vi "给选中行上色.vi"(4 "列数":i32, 6 "颜色":cluster{"未选中颜色盒":u32, "选中颜色盒":u32}={"未选中颜色盒"=16763272, "选中颜色盒"=12439011}, 8 "错误输入（无错误）":errorcluster, 9 "本次坐标":T1={"Row"=20, "Column"=20}, 10 "上次坐标":T1={"Row"=20, "Column"=20}, 11 "引用输入":refnum<vi>) -> (0 "错误输出":errorcluster, 2 "上次坐标输出":T1={"Row"=20, "Column"=20}, 3 "引用输出":refnum<vi>)   [LabVIEW 2014, in "表格.lvlib" / "表格上色.lvlib"]
uses:
  <vilib>/Utility/miscctls.llb/LVRowAndColumnTypeDef.ctl
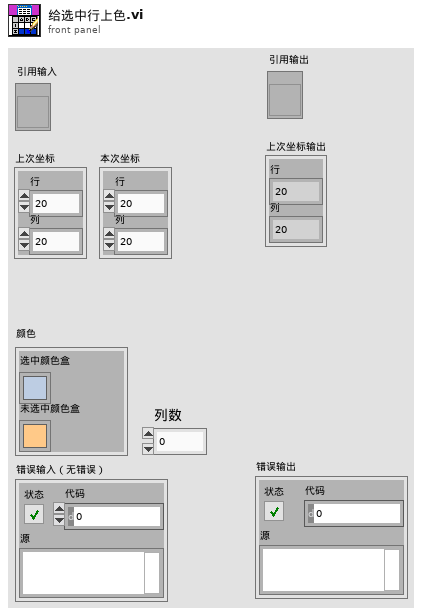
[diagram p1: front panel]
types:
  T1 = typedef "LVRowAndColumnTypeDef.ctl" = cluster{"Row":i32, "Column":i32}
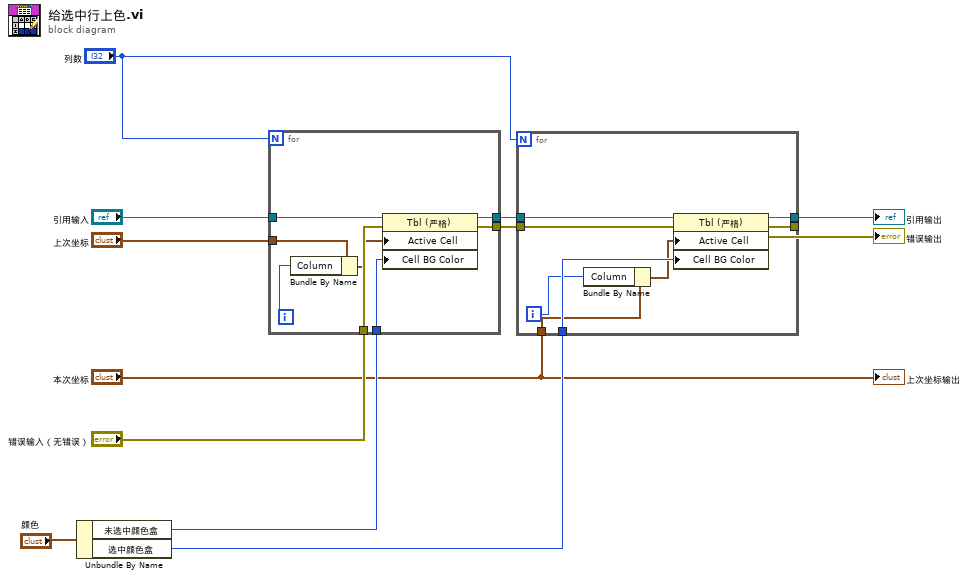
[diagram p0: block diagram]
diagram:
  n1 = Unbundle By Name("颜色") -> ("未选中颜色盒"=w11:u32, "选中颜色盒"=w10:u32)
  n2 = for {
    N: "列数" -> [_]
    tunnel: w11 -> [w20]
    tunnel: "错误输入（无错误）" -> [w19]
    tunnel: [w18] -> w5
    tunnel: [w17] -> w4
    tunnel: "引用输入" -> [w16]
    tunnel: "上次坐标" -> [w15]
    i -> [w14]
    n3 = Bundle By Name(cluster=w15, "Column"=w14) -> (w13:T1)
    n4 = property on="属性节点" class="Tbl (严格)"(reference=w16, error in=w19, "Active Cell"=w13, "Cell BG Color"=w20) -> (reference out=w18:refnum<vi>, error out=w17:errorcluster)
  }
  n5 = for {
    N: "列数" -> [_]
    tunnel: w10 -> [w28]
    tunnel: [w27] -> w8
    tunnel: "本次坐标" -> [w23]
    tunnel: [w26] -> w6
    tunnel: w5 -> [w25]
    tunnel: w4 -> [w24]
    i -> [w22]
    n6 = Bundle By Name(cluster=w23, "Column"=w22) -> (w21:T1)
    n7 = property on="属性节点" class="Tbl (严格)"(reference=w25, error in=w24, "Active Cell"=w21, "Cell BG Color"=w28) -> (reference out=w26:refnum<vi>, error out=w27:errorcluster)
  }
  "错误输出" <- w8
  "引用输出" <- w6
  "上次坐标输出" <- "本次坐标"
